vi "Profile Timer.vi"(2 "Label":string, 7 "error in (no error)":errorcluster, 13 "Timer Action (Start)":T2) -> (8 "error out":errorcluster, 14 "All Function Timestamps":T1[](array[typedef]))   [LabVIEW 2021]
uses:
  <vilib>/myRIO/Common/Express VI Framework/typedefs/Timer Action.ctl
  <vilib>/myRIO/Common/Express VI Framework/typedefs/Function Timestamp.ctl
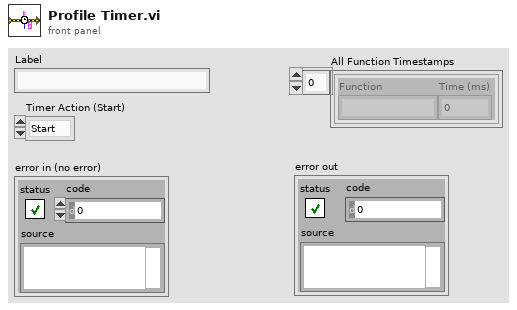
[diagram p1: front panel]
types:
  T1 = typedef "Function Timestamp.ctl" = cluster{"Function":string, "Time (ms)":u32}
  T2 = typedef "Timer Action.ctl" = enum16{"Start", "End", "Get All", "Clear All"}
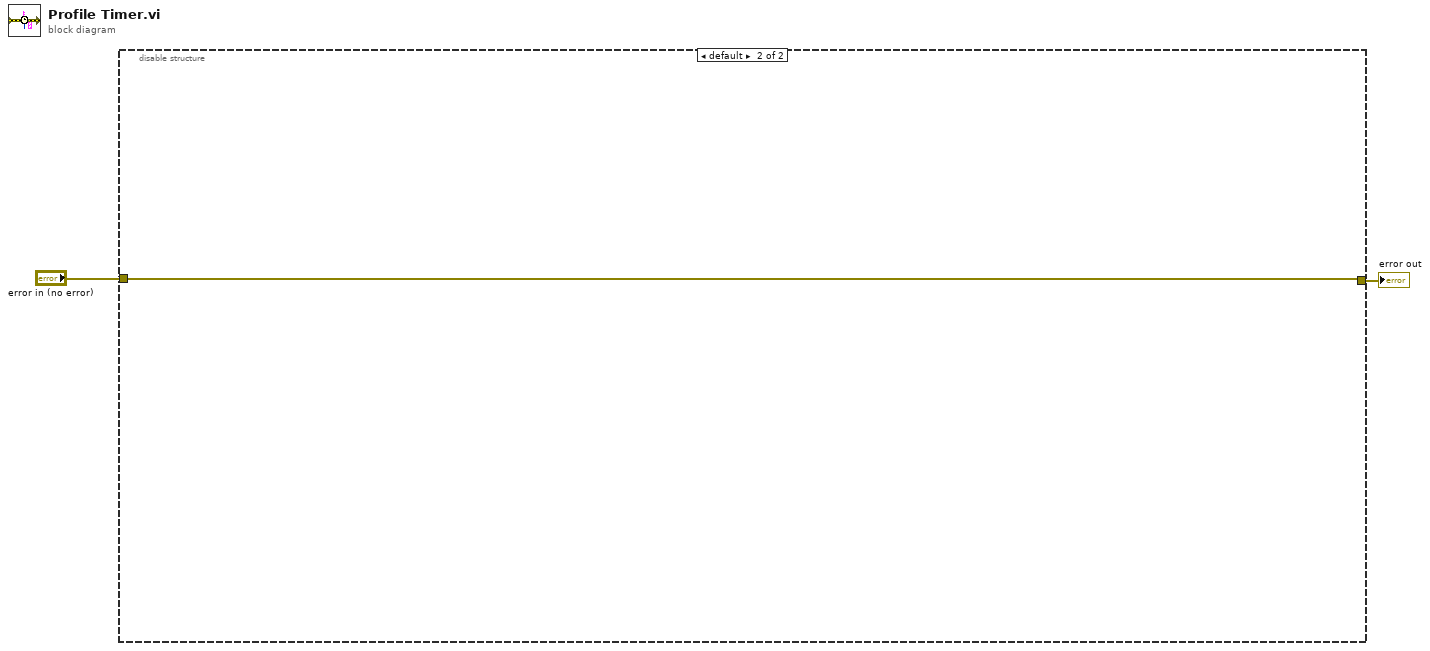
[diagram p0: block diagram]
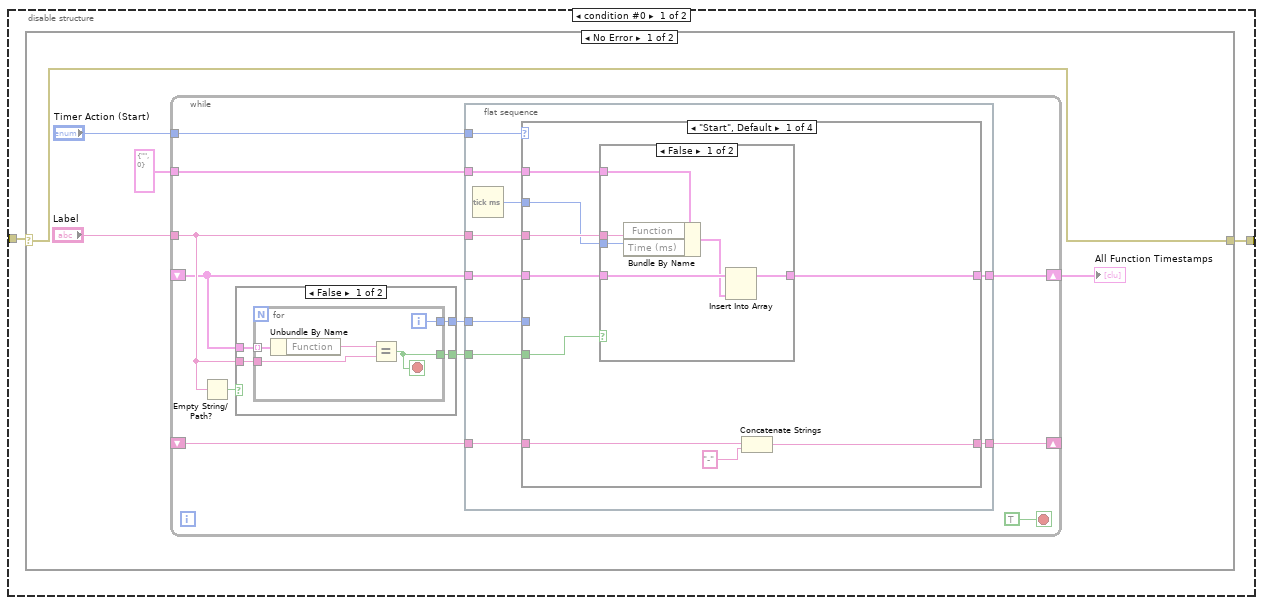
[diagram p2: hidden frame]
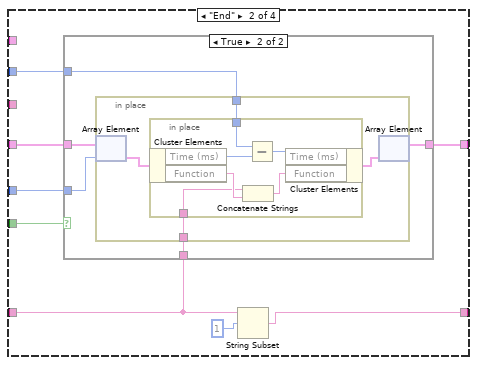
[diagram p4: hidden frame]
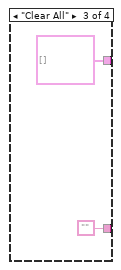
[diagram p6: hidden frame]
diagram:
  n1 = disable-structure shown="default" {
    disable-tunnel: "error in (no error)" -> [w4 w85]
    disable-tunnel: [w3 w85] -> w1
    frame condition #0 {
      n2 = case shown="No Error" w4 {
        selector: w4 -> [w5 w84]
        tunnel: [w5 w84] -> w3
        frame No Error {
          n3 = while {
            tunnel: "Label" -> [w15]
            tunnel: T1 {"Function"="", "Time (ms)"=0} -> [w20]
            tunnel: "Timer Action (Start)" -> [w19]
            shift-right: [w13] -> w6
            shift-left: _ -> [w12]
            shift-right: [w10] -> _
            shift-left: _ -> [w11]
            stop <- TRUE stop-if-true
            n4 = Empty String/Path?(string/path=w15) -> (empty?=w14:bool)
            n5 = case shown="False" w14 {
              tunnel: w12 -> [w78 _]
              tunnel: [w77 _] -> w18
              tunnel: [w76 _] -> w17
              tunnel: w15 -> [w75 _]
              frame False {
                n6 = for {
                  tunnel: w78 -> [w83] mode=indexing
                  tunnel: w75 -> [w81]
                  tunnel: [w80] -> w77
                  tunnel: [w79] -> w76
                  i -> [w79]
                  stop <- w80 stop-if-true
                  n7 = Unbundle By Name(w83) -> ("Function"=w82:string)
                  n8 = Equal?(x=w82, y=w81) -> (x = y?=w80:bool)
                }
              }
              frame True {
              }
            }
            n9 = flat-sequence {
              tunnel: w20 -> [w29]
              tunnel: w19 -> [w28]
              tunnel: w18 -> [w27]
              tunnel: w17 -> [w26]
              tunnel: w15 -> [w25]
              tunnel: [w24] -> w13
              tunnel: w12 -> [w23]
              tunnel: w11 -> [w22]
              tunnel: [w21] -> w10
              frame #0 {
                n10 = Tick Count (ms)() -> (millisecond timer value=w30:u32)
                n11 = case shown="\"Start\", Default" w28 {
                  tunnel: w30 -> [w36 w53 _ _]
                  tunnel: w23 -> [w39 w52 _ w74]
                  tunnel: w25 -> [w37 _ _ _]
                  tunnel: w29 -> [w38 _ _ _]
                  tunnel: [w35 w50 T1[] [] w74] -> w24
                  tunnel: w27 -> [w34 w54 _ _]
                  tunnel: w26 -> [_ w51 _ _]
                  tunnel: w22 -> [w32 w47 _ w73]
                  tunnel: [w31 w48 "" w73] -> w21
                  frame "Start", Default {
                    n12 = case shown="False" w34 {
                      tunnel: w39 -> [w45 w46]
                      tunnel: w38 -> [w44 _]
                      tunnel: w37 -> [w42 _]
                      tunnel: w36 -> [w41 _]
                      tunnel: [w40 w46] -> w35
                      frame False {
                        n13 = Bundle By Name(cluster=w44, "Function"=w42, "Time (ms)"=w41) -> (w43:T1)
                        n14 = Insert Into Array(array=w45, new element=w43) -> (w40:T1[])  [unwired: 1 in]
                      }
                      frame True {
                      }
                    }
                    n15 = Concatenate Strings(w32, "-" ("string")) -> (w31:string)
                  }
                  frame "End" {
                    n16 = case shown="True" w54 {
                      tunnel: w53 -> [_ w58]
                      tunnel: w52 -> [w55 w60]
                      tunnel: w51 -> [_ w59]
                      tunnel: [w55 w57] -> w50
                      tunnel: w47 -> [_ w56]
                      frame False {
                      }
                      frame True {
                        n17 = in-place {
                          in-place-border: w58 -> [w64]
                          in-place-border: w56 -> [w61]
                          n18 = in-place-array #1(w60, w59) -> (w63:T1)
                          n19 = in-place {
                            in-place-border: w64 -> [w70]
                            in-place-border: w61 -> [w65]
                            n20 = in-place-cluster #2(w63) -> ("Time (ms)"=w69:u32, "Function"=w66:string)
                            n21 = Concatenate Strings(w65, w66) -> (w67:string)
                            n22 = Subtract(x=w70, y=w69) -> (x-y=w68:u32)
                            n23 = in-place-cluster #2("Time (ms)"=w68, "Function"=w67) -> (w62:T1)
                          }
                          n24 = in-place-array #1(w62) -> (w57:T1[])  [unwired: 1 out]
                        }
                      }
                    }
                    n25 = String Subset(string=w47, offset (0)=1) -> (substring=w48:string)  [unwired: 1 in]
                  }
                  frame "Clear All" {
                  }
                  frame "Get All" {
                  }
                }
              }
            }
          }
          "All Function Timestamps" <- w6
        }
        frame Error {
        }
      }
    }
    frame condition #1 (active) {
    }
  }
  "error out" <- w1
